vi "15_5_Fxp_addation.vi"(1 "y":fxp<+/-,5,15>, 2 "x":fxp<+/-,5,15>) -> (0 "x+y":fxp<+/-,6,16> format="%.41g")   [LabVIEW 2020]
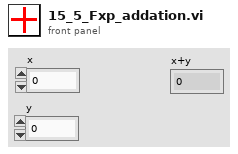
[diagram p1: front panel]
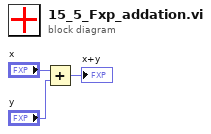
[diagram p0: block diagram]
diagram:
  n1 = Add(x="x", y="y") -> (x+y=→"x+y":fxp<+/-,6,16>)
